vi "FilePath.vi"(11 "Boolean":bool) -> (3 "Path":path)   [LabVIEW 2015]
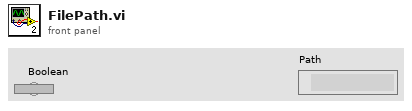
[diagram p1: front panel]
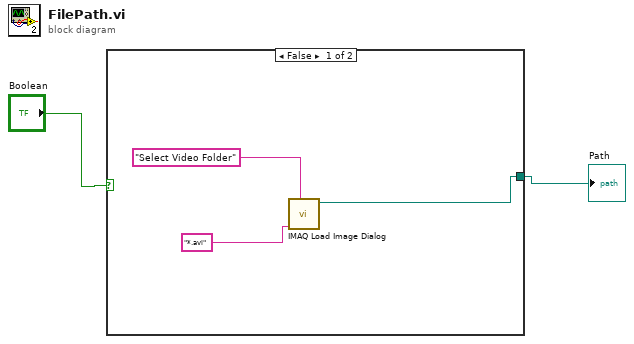
[diagram p0: block diagram]
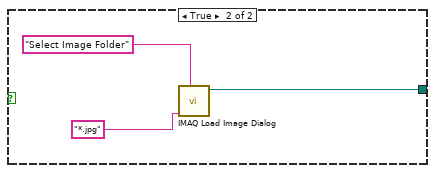
[diagram p2: hidden frame]
diagram:
  n1 = case shown="False" "Boolean" {
    tunnel: [w3 w6] -> w1
    frame False {
      n2 = call "IMAQ Load Image Dialog"("Prompt"="Select Video Folder", "Pattern"="*.avi") -> ("Path"=w3:path)  [unwired: 7 in, 2 out]
    }
    frame True {
      n3 = call "IMAQ Load Image Dialog"("Prompt"="Select Image Folder", "Pattern"="*.jpg") -> ("Path"=w6:path)  [unwired: 7 in, 2 out]
    }
  }
  "Path" <- w1
